vi "XNET String To IO Name (Subframe).vi"(3 "string":string) -> (0 "XNET Subframe":refnum<k21>)   [LabVIEW 2018]
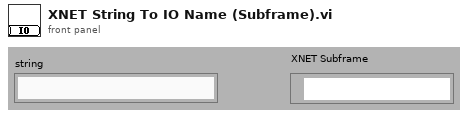
[diagram p1: front panel]
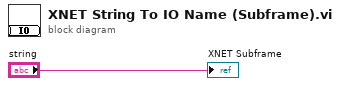
[diagram p0: block diagram]
diagram:
  "XNET Subframe" <- "string"
